vi "rename Class Input Output.vi"() -> ()   [LabVIEW 2020]
doc: "Mit Hilfe dieses VI lassen sich die Namen der LabViewClassControls ändern. Das VI zeigt eine Liste von gefundenen Control-Namen und markiert die zu ändernden Control-Namen entsprechend der Einstellungen des Benutzers für [Pattern] und [Replace String]. Der Benutzer hat die Möglichkeit die Auswahl zu änden (CTRL-Taste drücken und gewünschte Elemente dazu- oder wegnehmen). Auf Knopfdruck ([rename selected]) werden die ausgewählten Control-Namen geändert."
panel:
  in  "rename":bool
  in  "Replace String":string
  in  "Pattern":string
  in  "Project list":i32(listbox)
  in  "stop":bool
  in  "mlb":i32[](listbox)
  # "Instruction for use:\n1. Select VIs to rename in Project Explorer\n2. Start program and select the Project from the project list\n3. Enter a search pattern and VIs with class terminal labels matching the pattern are high-lighted\n4. Enter a replacement string, check the new name preview and then press \"rename selected\" to actually rename.\n5. Repeat steps 3 and 4 for additional renaming. Restart program to rename other VIs."
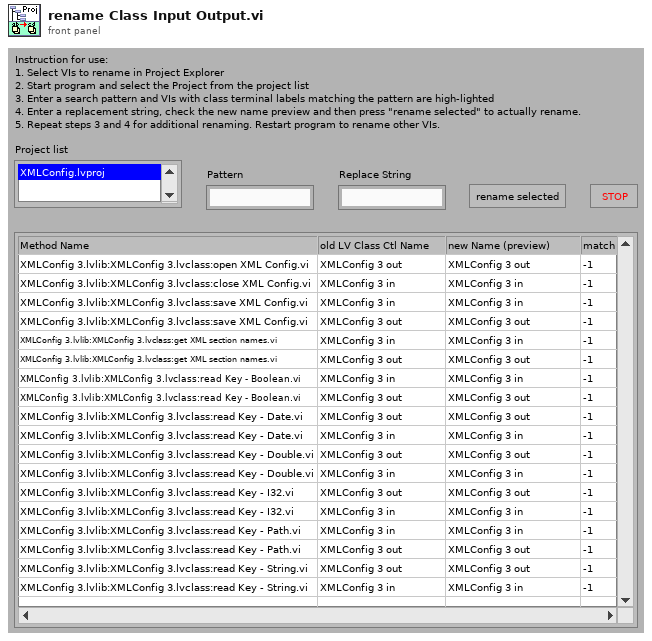
[diagram p1: front panel]
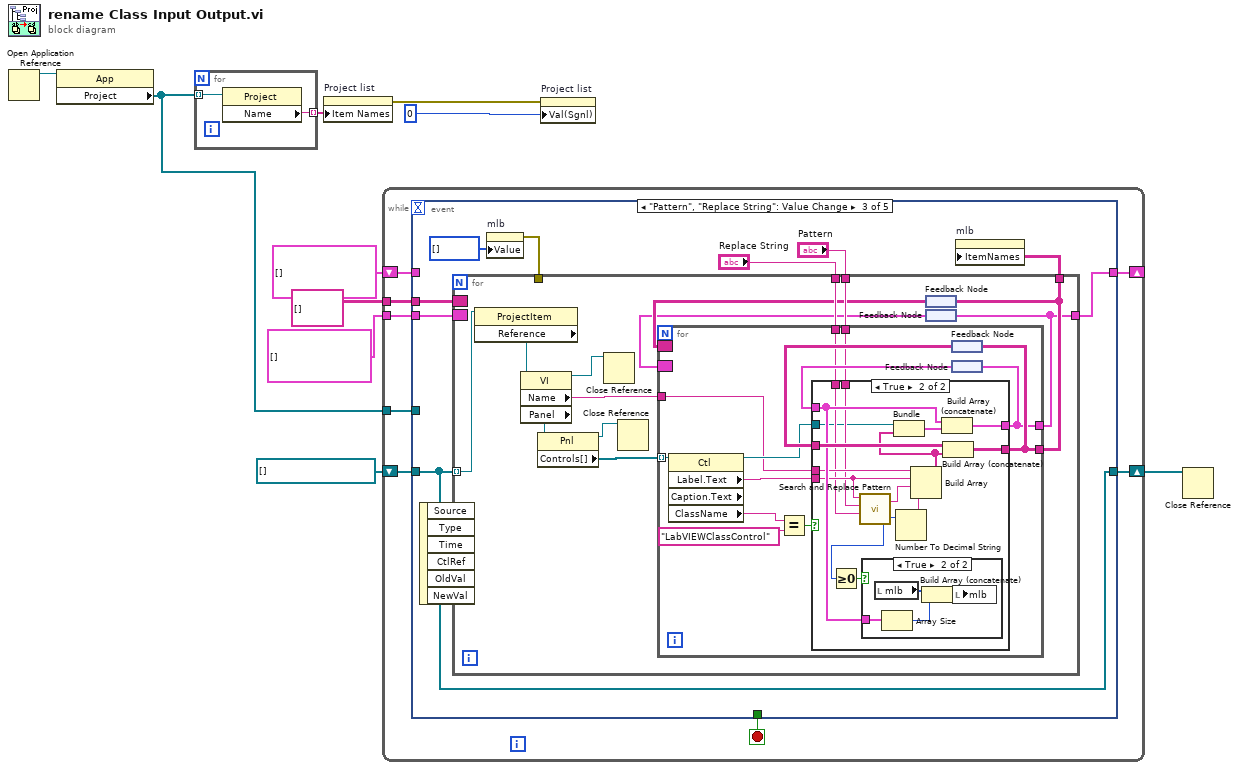
[diagram p0: block diagram]
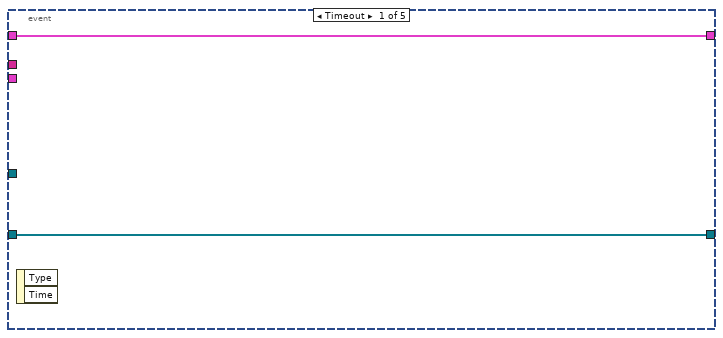
[diagram p2: hidden frame]
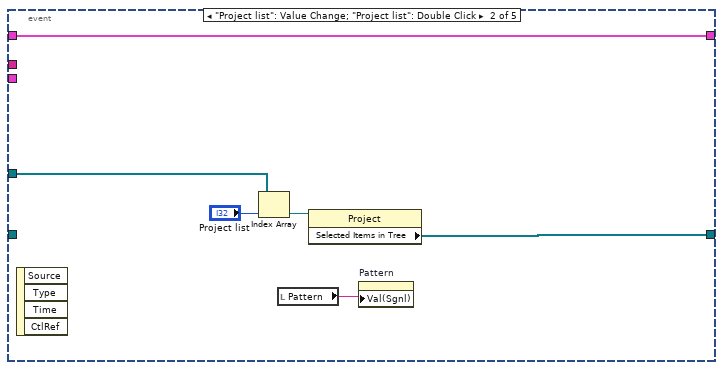
[diagram p3: hidden frame]
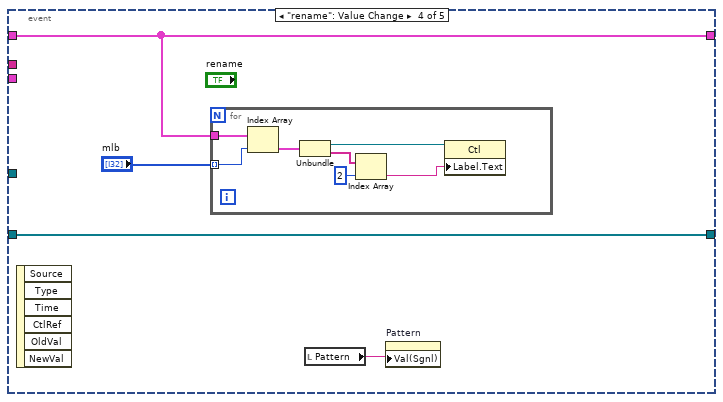
[diagram p6: hidden frame]
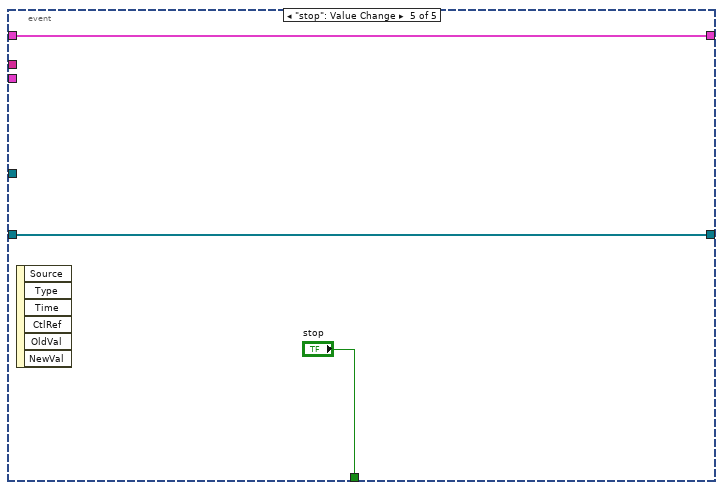
[diagram p7: hidden frame]
diagram:
  n1 = Open Application Reference() -> (3:w10:refnum<vi>)  [unwired: 1 in, 4 out]
  n2 = property class="App"(reference=w10) -> ("Project"=w8:refnum<vi>[])  [unwired: 1 in, 2 out]
  n3 = for {
    tunnel: w8 -> [w12] mode=indexing
    tunnel: [w11] -> w9 mode=indexing
    n4 = property class="Project"(reference=w12) -> ("Name"=w11:string)  [unwired: 1 in, 2 out]
  }
  n5 = property on="Project list" class="LstBox (strict)"("Item Names"=w9) -> (error out=w7:errorcluster)  [unwired: 2 in, 1 out]
  n6 = while {
    shift-right: [w18] -> w4
    shift-left: refnum<vi>[] [] ("Selected Items in Tree") -> [w17]
    tunnel: w8 -> [w19]
    shift-right: [w16] -> _
    shift-left: cluster{refnum<vi>, string[]}[] [] -> [w15]
    tunnel: string[][] [] -> [w14]
    tunnel: cluster{refnum<vi>, string[]}[] [] -> [w13]
    stop <- w20 stop-if-true
    n7 = event shown="[2] \"Pattern\", \"Replace String\": Value Change" {
      selector: _ -> [_ _ _ _ _]
      dyn-events: _ -> [_ _ _ _ _]
      timeout: _ -> [_ _ _ _ _]
      tunnel: [_ _ _ _ "stop"] -> w20
      tunnel: w19 -> [_ w26 _ _ _]
      tunnel: [w22 w25 w37 w87 w97] -> w18
      tunnel: w17 -> [w22 _ w37 w87 w97]
      tunnel: [w21 w23 w32 w86 w96] -> w16
      tunnel: w15 -> [w21 w23 _ w86 w96]
      tunnel: w14 -> [_ _ w34 _ _]
      tunnel: w13 -> [_ _ w33 _ _]
      event Timeout {
        n8 = event-data() -> ()  [unwired: 3 out]
      }
      event "Project list": Value Change; "Project list": Double Click {
        n9 = event-data() -> ()  [unwired: 5 out]
        n10 = Index Array(array=w26, index="Project list") -> (element=w28:refnum<vi>)
        n11 = local read "Pattern"() -> (w24:string)
        n12 = property class="Project"(reference=w28) -> ("Selected Items in Tree"=w25:refnum<vi>[])  [unwired: 1 in, 2 out]
        n13 = property on="Pattern" class="Str"("Val(Sgnl)"=w24) -> ()  [unwired: 2 in, 2 out]
      }
      event "Pattern", "Replace String": Value Change {
        n14 = event-data() -> ()  [unwired: 7 out]
        n15 = property on="mlb" class="MCListbox (strict)"("Value"=i32[] [] ("mlb")) -> (error out=w29:errorcluster)  [unwired: 2 in, 1 out]
        n16 = for {
          tunnel: w37 -> [w49] mode=indexing
          tunnel: "Pattern" -> [w48]
          tunnel: "Replace String" -> [w47]
          border: w34 -> [_]
          tunnel: [w43] -> w31
          border: w33 -> [_]
          tunnel: [w39] -> w32
          tunnel: w29 -> [_]
          n17 = property class="ProjectItem"(reference=w49) -> ("Reference"=w50:refnum<vi>)  [unwired: 1 in, 2 out]
          n18 = property class="VI"(reference=w50) -> (reference out=w38:refnum<vi>, "Name"=w45:string, "Panel"=w46:refnum<vi>)  [unwired: 1 in, 1 out]
          n19 = property class="Pnl"(reference=w46) -> (reference out=w41:refnum<vi>, "Controls[]"=w42:refnum<vi>[])  [unwired: 1 in, 1 out]
          n20 = Close Reference(reference=w38) -> ()  [unwired: 1 in, 1 out]
          n21 = Close Reference(reference=w41) -> ()  [unwired: 1 in, 1 out]
          n22 = feedback #1() -> (w44:string[][])
          n23 = feedback #2() -> (w40:cluster{refnum<vi>, string[]}[])
          n24 = for {
            tunnel: w42 -> [w63] mode=indexing
            tunnel: [w59] -> w43
            border: w44 -> [_]
            border: w40 -> [_]
            tunnel: [w55] -> w39
            tunnel: w48 -> [w51]
            tunnel: w47 -> [w52]
            tunnel: w45 -> [w53]
            n25 = property class="Ctl" props=["Label", "Text", "Caption", "Text", "ClassName"](reference=w63) -> (reference out=w57:refnum<vi>, "Label.Text"=w54:string, "ClassName"=w61:string)  [unwired: 1 in, 2 out]
            n26 = Equal?(x=w61, y="LabVIEWClassControl") -> (x = y?=w60:bool)
            n27 = feedback #3() -> (w58:string[][])
            n28 = feedback #4() -> (w56:cluster{refnum<vi>, string[]}[])
            n29 = case shown="True" w60 {
              tunnel: w54 -> [_ w75]
              tunnel: [w65 w71] -> w59
              tunnel: w58 -> [w65 w80]
              tunnel: w57 -> [_ w69]
              tunnel: [w64 w78] -> w55
              tunnel: w56 -> [w64 w79]
              tunnel: w53 -> [_ w77]
              tunnel: w52 -> [_ w74]
              tunnel: w51 -> [_ w73]
              frame False {
              }
              frame True {
                n30 = call <vilib>:"Search and Replace Pattern.vi"("string"=w75, "regular expression (\"\")"=w73, "replace string (\"\")"=w74) -> ("result string"=w76:string, "offset past match"=w67:i32)  [unwired: 2 out]
                n31 = Greater Or Equal To 0?(x=w67) -> (x >= 0?=w66:bool)
                n32 = case shown="True" w66 {
                  tunnel: w79 -> [_ w81]
                  frame False {
                  }
                  frame True {
                    n33 = local read "mlb"() -> (w83:i32[])
                    n34 = Array Size(array=w81) -> (size(s)=w82:i32)
                    n35 = Build Array (concatenate)(w83, w82) -> (w84:i32[])
                    n36 = local write "mlb"(w84) -> ()
                  }
                }
                n37 = Number To Decimal String(number=w67) -> (decimal integer string=w72:string)  [unwired: 1 out]
                n38 = Build Array(w77, w75, w76, w72) -> (w70:string[])
                n39 = Bundle(w69, w70) -> (w68:cluster{refnum<vi>, string[]})  [unwired: 1 out]
                n40 = Build Array (concatenate)(w79, w68) -> (w78:cluster{refnum<vi>, string[]}[])
                n41 = Build Array (concatenate)(w80, w70) -> (w71:string[][])
              }
            }
            n42 = feedback-in #3(w59) -> ()
            n43 = feedback-in #4(w55) -> ()
          }
          n44 = feedback-in #1(w43) -> ()
          n45 = feedback-in #2(w39) -> ()
        }
        n46 = property on="mlb" class="MCListbox (strict)"("ItemNames"=w31) -> ()  [unwired: 2 in, 2 out]
      }
      event "rename": Value Change {
        n47 = event-data() -> ()  [unwired: 7 out]
        n48 = for {
          tunnel: "mlb" -> [w94] mode=indexing
          tunnel: w86 -> [w95]
          n49 = Index Array(array=w95, index=w94) -> (element=w93:cluster{refnum<vi>, string[]})
          n50 = Unbundle(w93) -> (w92:refnum<vi>, w91:string[])
          n51 = Index Array(array=w91, index=2) -> (element=w89:string)
          n52 = property class="Ctl"(reference=w92, "Label.Text"=w89) -> ()  [unwired: 1 in, 2 out]
        }
        n53 = local read "Pattern"() -> (w85:string)
        n54 = property on="Pattern" class="Str"("Val(Sgnl)"=w85) -> ()  [unwired: 2 in, 2 out]
      }
      event "stop": Value Change {
        n55 = event-data() -> ()  [unwired: 7 out]
      }
    }
  }
  n56 = property on="Project list" class="LstBox (strict)"(error in=w7, "Val(Sgnl)"=0 ("Value (Signaling)")) -> ()  [unwired: 1 in, 2 out]
  n57 = Close Reference(reference=w4) -> ()  [unwired: 1 in, 1 out]
